vi "Fault Handling.vi"(8 "error in":errorcluster, 10 "FaultCode":i32, 11 "PostUUT in":refnum<class "PostUUT.lvclass">) -> (0 "error out":errorcluster, 2 "Fault codes":cluster{"Bit":string, "Description":string}[](array[cluster]), 3 "PostUUT out":refnum<class "PostUUT.lvclass">)   [LabVIEW 2021, in "OPC UA.lvlib" / "PostUUT.lvclass"]
uses:
  PostUUT.lvclass
  PostUUT.lvclass/PostUUT.ctl
  OPC UA/OPC UA.lvclass
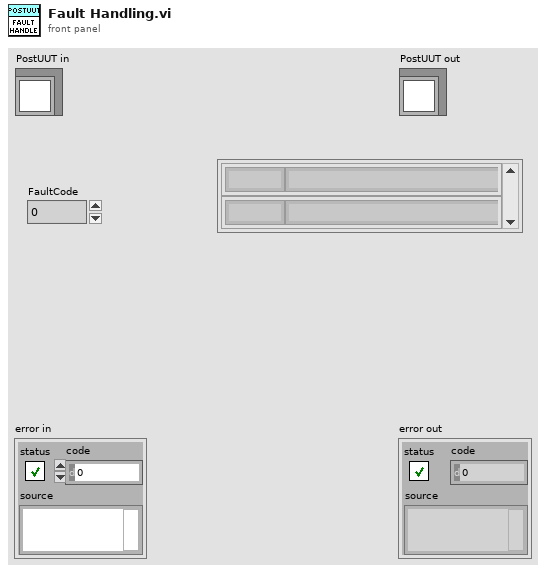
[diagram p1: front panel]
types:
  T1 = typedef "PostUUT.lvclass/Rx PostUUT.ctl" = cluster{"ResultsAck":bool, "Reset":bool, "Stop":bool, "FaultCode":u32}
  T2 = typedef "PostUUT.lvclass/Tx PostUUT.ctl" = cluster{"ResultsReady":bool, "Results":u32, "ElapsedTime":i32, "TimeCompleted":i32[], "Fault":bool, "Timeout":bool}
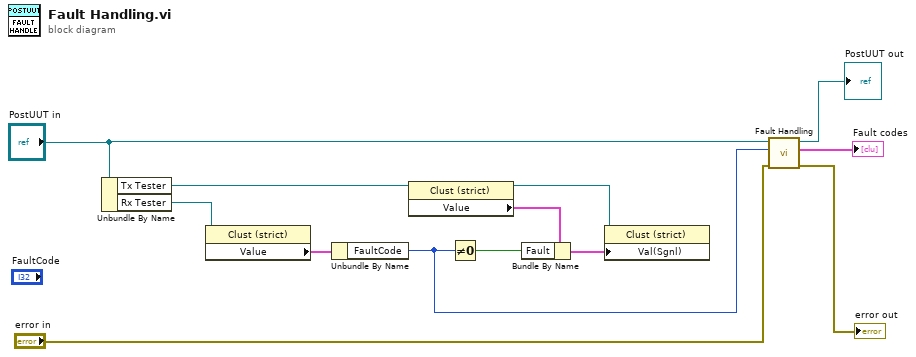
[diagram p0: block diagram]
diagram:
  n1 = Unbundle By Name("PostUUT in") -> ("Tx Tester"=w8:refnum<vi>, "Rx Tester"=w6:refnum<vi>)
  n2 = property class="Clust (strict)"(reference=w6) -> ("Value"=w7:T1)  [unwired: 1 in, 2 out]
  n3 = Unbundle By Name(w7) -> ("FaultCode"=w4:u32)
  n4 = property class="Clust (strict)"(reference=w8) -> (reference out=w11:refnum<vi>, "Value"=w9:T2)  [unwired: 1 in, 1 out]
  n5 = Not Equal To 0?(x=w4) -> (x != 0?=w3:bool)
  n6 = Bundle By Name(cluster=w9, "Fault"=w3) -> (w10:T2)
  n7 = property class="Clust (strict)"(reference=w11, "Val(Sgnl)"=w10) -> ()  [unwired: 1 in, 2 out]
  n8 = call-parent "Fault Handling.vi"("error in (no error)"="error in", "FaultCode"=w4, "OPC UA in"="PostUUT in") -> ("error out"=→"error out":errorcluster, "Fault codes"=→"Fault codes":cluster{"Bit":string, "Description":string}[], "OPC UA out"=→"PostUUT out":refnum<class "PostUUT.lvclass">)  [unwired: 6 in]
